vi "GetLVObject.vi"(8 "error in (no error)":errorcluster, 9 "StructuredData in":variant, 10 "Object Type":refnum<class>, 11 "BlueSerializer in":refnum<class "BlueSerializer.lvclass">) -> (0 "error out":errorcluster, 1 "StructuredData out":variant, 2 "Object out":refnum<class>, 3 "BlueSerializer out":refnum<class "BlueSerializer.lvclass">)   [LabVIEW 2019, in "BlueSerialization.lvlib" / "BlueSerializer.lvclass"]
uses:
  BlueSerializer.lvclass
  BlueSerializer.lvclass/BlueSerializer.ctl
  BlueSerializable/BlueSerializable.lvclass
  Support/SetSerializableDataCluster.ctl
  Support/SetSerializableDataClusterIterable.ctl
  Support/SetSerializableDataClusterLayer.ctl
  BlueSerializableVersion.ctl
  Support/SetSerializableDataObject.ctl
  FindMutationByVerIndex.vi
  MutationParentLevelsRemoved.vi
  MutationParentLevelsAdded.vi
  MutationOptionsErrorCheck.vi
  SliceClass.vi
  <resource>/Framework/Providers/BlueSerializationProviderShared/GetVersionNumberFromMutation.vi
  <resource>/Framework/Providers/BlueSerializationProviderShared/FindMutationHistoryIndex.vi
  <resource>/Framework/Providers/BlueSerializationProviderShared/UserCommentToVersion.vi
  <vilib>/Utility/error.llb/Error Cluster From Error Code.vi
  <vilib>/Utility/LVClass/Get LV Class Default Value By Name.vi
  DeserializeInitTargetObjectAndStack.vi
  <vilib>/Utility/EditLVLibs/LVClass/Get Mutation History.vi
  <vilib>/ErrorRing/Error Ring.xnode
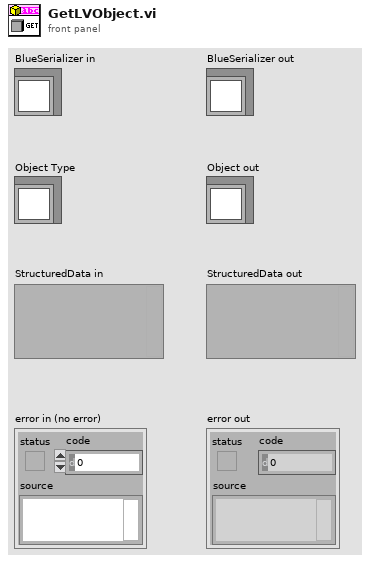
[diagram p1: front panel]
types:
  T1 = typedef "BlueSerialization.lvlib/BlueSerializer.lvclass/DeserializeOptions.ctl" = cluster{"deserialize non-BlueSerializable objects from hex?":bool, "expand objects on type conflict?":bool, "Slicing":T2, "Mutation Options":T3, "Preservation Options":T4}
  T2 = typedef "BlueSerialization.lvlib/BlueSerializer.lvclass/DeserializeSlicingOptions.ctl" = cluster{"slice flattened object data on error?":bool, "sliceable class names":string[]}
  T3 = typedef "BlueSerialization.lvlib/BlueSerializer.lvclass/DeserializeMutationOptions.ctl" = cluster{"error on inserted parent levels?":bool, "\terror on obsolete parent levels?":bool}
  T4 = typedef "BlueSerialization.lvlib/BlueSerializer.lvclass/DeserializePreservationOptions.ctl" = cluster{"Preserve wired non-serialized data?":bool, "Preserve wired serialized data?":bool}
  T5 = typedef "BlueSerialization.lvlib/BlueSerializer.lvclass/ClassHeader.ctl" = cluster{"Class Name":string, "Library Version":T6, "default data?":bool}
  T6 = typedef "Edit LVLibs.lvlib/LibVersion.ctl" = cluster{"Major":u16, "Minor":u16, "Fix":u16, "Build":u16}
  T7 = typedef "BlueSerialization.lvlib/BlueSerializer.lvclass/SetSerializableDataCluster.ctl" = cluster{"StructuredData":variant, "ClassOps (child, parent)":T8[]}
  T8 = typedef "BlueSerialization.lvlib/BlueSerializer.lvclass/SetSerializableDataClusterIterable.ctl" = cluster{"Layer":T9, "SerializedClassName":string, "default data?":bool, "BlueSerializableVersion":T10, "object":T11}
  T9 = typedef "BlueSerialization.lvlib/BlueSerializer.lvclass/SetSerializableDataClusterLayer.ctl" = enum16{"new class layer", "dropped class layer", "agreed class layer"}
  T10 = typedef "BlueSerialization.lvlib/BlueSerializer.lvclass/BlueSerializableVersion.ctl" = cluster{"From":u16, "To":u16}
  T11 = typedef "BlueSerialization.lvlib/BlueSerializer.lvclass/SetSerializableDataObject.ctl" = cluster{"default object":refnum<class "BlueSerializable.lvclass">, "SerializableDataOverride":variant, "UseSerializableDataOverride?":bool}
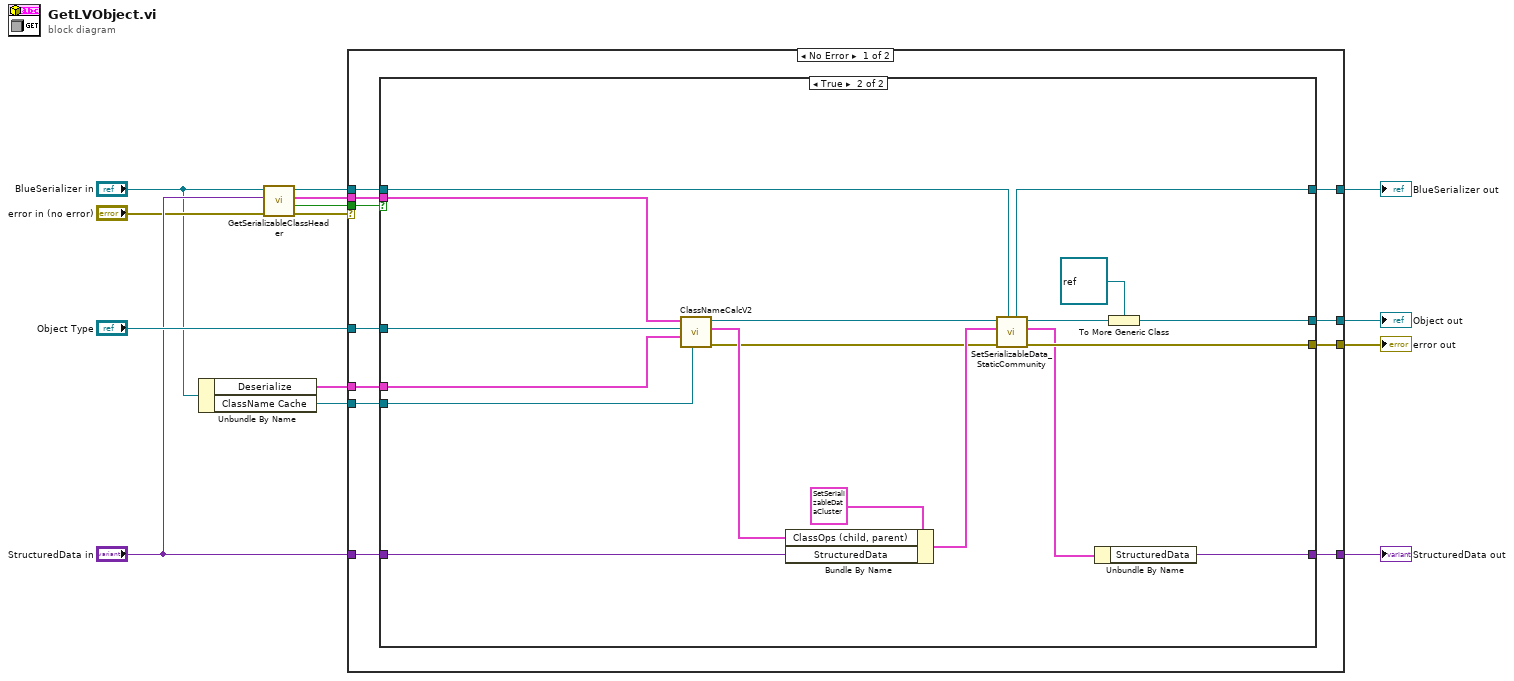
[diagram p0: block diagram]
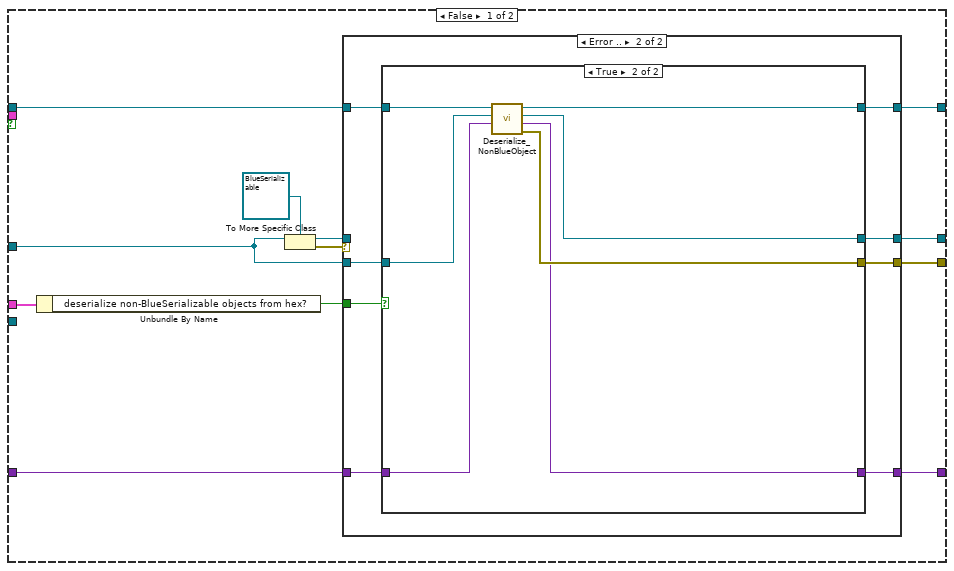
[diagram p2: hidden frame]
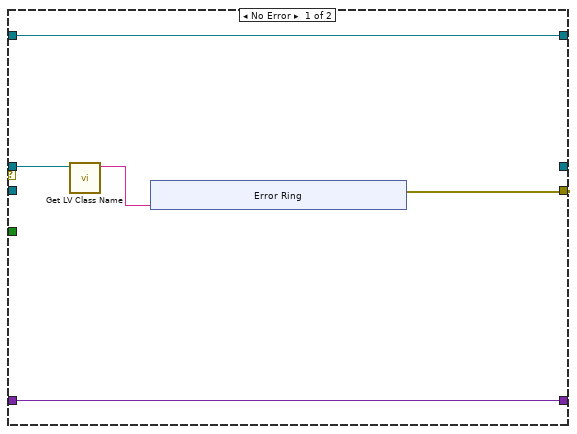
[diagram p3: hidden frame]
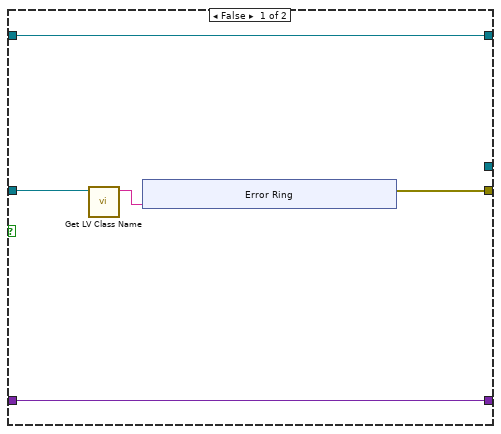
[diagram p4: hidden frame]
diagram:
  n1 = Unbundle By Name("BlueSerializer in") -> ("Deserialize"=w3:T1, "ClassName Cache"=w2:refnum<data-value>)
  n2 = call "GetSerializableClassHeader.vi"("error in (no error)"="error in (no error)", "StructuredData"="StructuredData in", "BlueSerializer in"="BlueSerializer in") -> ("error out"=w6:errorcluster, "header found?"=w9:bool, "SerializedClassHeader (child,parent)"=w7:T5[], "BlueSerializer out"=w8:refnum<class "BlueSerializer.lvclass">)  [unwired: 5 in]
  n3 = case shown="No Error" w6 {
    selector: w6 -> [_ w96]
    tunnel: [w25 w97] -> w14
    tunnel: [w24 w96] -> w13
    tunnel: [w23 _] -> w12
    tunnel: "Object Type" -> [w22 _]
    tunnel: "StructuredData in" -> [w21 w95]
    tunnel: w9 -> [w20 _]
    tunnel: w8 -> [w19 w97]
    tunnel: w3 -> [w18 _]
    tunnel: w7 -> [w17 _]
    tunnel: w2 -> [w16 _]
    tunnel: [w15 w95] -> w5
    frame No Error {
      n4 = case shown="True" w20 {
        tunnel: [w30 w77] -> w25
        tunnel: [w34 w81] -> w24
        tunnel: [w31 w94] -> w23
        tunnel: w19 -> [w32 w78]
        tunnel: w21 -> [w29 w93]
        tunnel: w22 -> [w33 w87]
        tunnel: w18 -> [w27 w90]
        tunnel: w17 -> [_ w89]
        tunnel: w16 -> [_ w88]
        tunnel: [w28 w85] -> w15
        frame False {
          n5 = Unbundle By Name(w27) -> ("deserialize non-BlueSerializable objects from hex?"=w26:bool)
          n6 = To More Specific Class(target class=refnum<class "BlueSerializable.lvclass"> refnum ("BlueSerializer.lvlib:BlueSerializable.lvclass"), reference=w33) -> (specific class reference=w35:refnum<class "BlueSerializable.lvclass">, error out=w36:errorcluster)  [unwired: 1 in]
          n7 = case shown="Error .." w36 {
            tunnel: w35 -> [w42 _]
            tunnel: [w40 w52] -> w34
            tunnel: w33 -> [_ w57]
            tunnel: w29 -> [w38 w56]
            tunnel: w32 -> [w39 w55]
            tunnel: [_ w54] -> w31
            tunnel: w26 -> [_ w53]
            tunnel: [w39 w51] -> w30
            tunnel: [w38 w50] -> w28
            frame No Error {
              n8 = call <vilib>:"Get LV Class Name.vi"("object"=w42) -> ("class name"=w41:string)  [unwired: 9 in, 1 out]
              n9 = xnode "Error Ring"("parameter 0"=w41) -> ("error out"=w40:errorcluster)
            }
            frame Error {
              n10 = case shown="True" w53 {
                tunnel: w57 -> [w61 w74]
                tunnel: w56 -> [w58 w73]
                tunnel: w55 -> [w59 w76]
                tunnel: [_ w71] -> w54
                tunnel: [w62 w72] -> w52
                tunnel: [w59 w75] -> w51
                tunnel: [w58 w70] -> w50
                frame False {
                  n11 = call <vilib>:"Get LV Class Name.vi"("object"=w61) -> ("class name"=w60:string)  [unwired: 9 in, 1 out]
                  n12 = xnode "Error Ring"("parameter 0"=w60) -> ("error out"=w62:errorcluster)
                }
                frame True {
                  n13 = call "Deserialize_NonBlueObject.vi"("StructuredData in"=w73, "Object Type"=w74, "BlueSerializer in"=w76) -> ("error out"=w72:errorcluster, "StructuredData out"=w70:variant, "Object out"=w71:refnum<class>, "BlueSerializer out"=w75:refnum<class "BlueSerializer.lvclass">)  [unwired: 5 in]
                }
              }
            }
          }
        }
        frame True {
          n14 = call "ClassNameCalcV2.vi"("ClassName Cache"=w88, "Deserialize"=w90, "wired object"=w87, "SerializedClassHeader (child,parent)"=w89) -> ("error out"=w82:errorcluster, "ClassOps (child, parent)"=w86:T8[], "Target Object"=w84:refnum<class "BlueSerializable.lvclass">)  [unwired: 5 in]
          n15 = Bundle By Name(cluster=T7 {"StructuredData"=variant(string ""), "ClassOps (child, parent)"=[]} ("Cluster"), "ClassOps (child, parent)"=w86, "StructuredData"=w93) -> (w83:T7)
          n16 = call "SetSerializableData_StaticCommunity.vi"("BlueSerializer in"=w78, "error in (no error)"=w82, "Data In"=w83, "BlueSerializable in"=w84) -> ("error out"=w81:errorcluster, "Data Out"=w80:T7, "BlueSerializable out"=w79:refnum<class "BlueSerializable.lvclass">, "BlueSerializer out"=w77:refnum<class "BlueSerializer.lvclass">)  [unwired: 4 in]
          n17 = Unbundle By Name(w80) -> ("StructuredData"=w85:variant)
          n18 = To More Generic Class(target class=refnum<class> refnum ("Object out"), reference=w79) -> (generic class reference=w94:refnum<class>)
        }
      }
    }
    frame Error {
    }
  }
  "error out" <- w13
  "BlueSerializer out" <- w14
  "Object out" <- w12
  "StructuredData out" <- w5
